vi "Grid_RandomMapping.vi"(10 "Point":i64, 11 "NumPoints":i64=64000) -> (3 "element":i64=42888)   [LabVIEW 2014]
panel:
  out "Run":bool
  out "Randomized Array":i64[](array[numeric])
  out "Array":i32[](array[numeric])
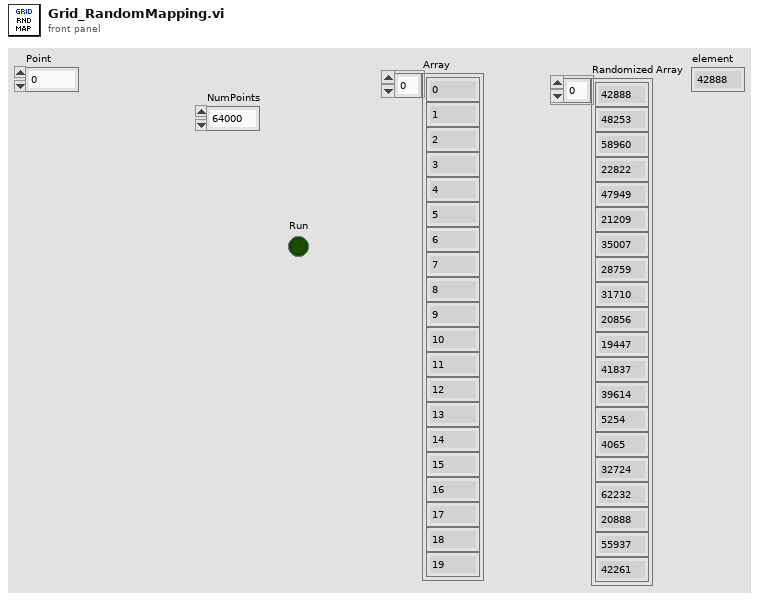
[diagram p1: front panel]
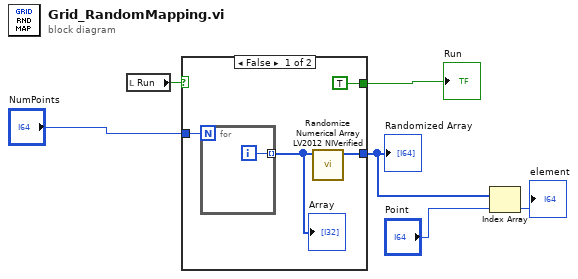
[diagram p0: block diagram]
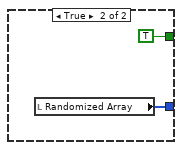
[diagram p2: hidden frame]
diagram:
  n1 = local read "Run"() -> (w4:bool)
  n2 = case shown="False" w4 {
    tunnel: "NumPoints" -> [w10 _]
    tunnel: [w8 w13] -> w2
    tunnel: [TRUE ("Run") TRUE ("Run")] -> w5
    frame False {
      n3 = for {
        N: w10 -> [_]
        tunnel: [w11] -> w9 mode=indexing
        i -> [w11]
      }
      "Array" <- w9
      n4 = call "Randomize Numerical Array LV2012 NIVerified.vi"("Array"=w9) -> ("Randomized Array"=w8:i64[])  [unwired: 10 in]
    }
    frame True {
      n5 = local read "Randomized Array"() -> (w13:i64[])
    }
  }
  "Randomized Array" <- w2
  "Run" <- w5
  n6 = Index Array(array=w2, index="Point") -> (element=→"element":i64)
